vi "_caraya_updateVInames.vi"(8 "error in (no error)":errorcluster, 10 "Application":refnum<vi>, 11 "Class Path":path=path "C:/Projects/JKI/Caraya/src/tests/test-all-asserts/Test Runner.AllAsserts.lvclass") -> (0 "error out":errorcluster)   [LabVIEW 2013]
uses:
  <vilib>/regexp/Match Regular Expression.xnode
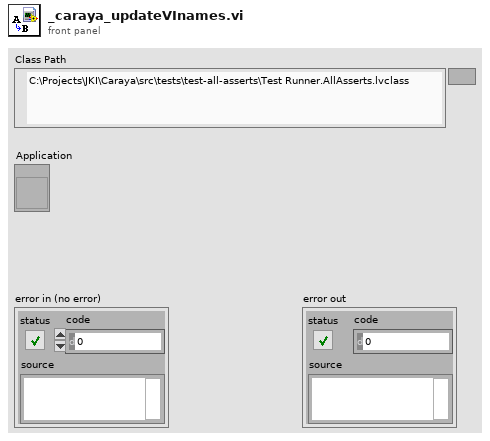
[diagram p1: front panel]
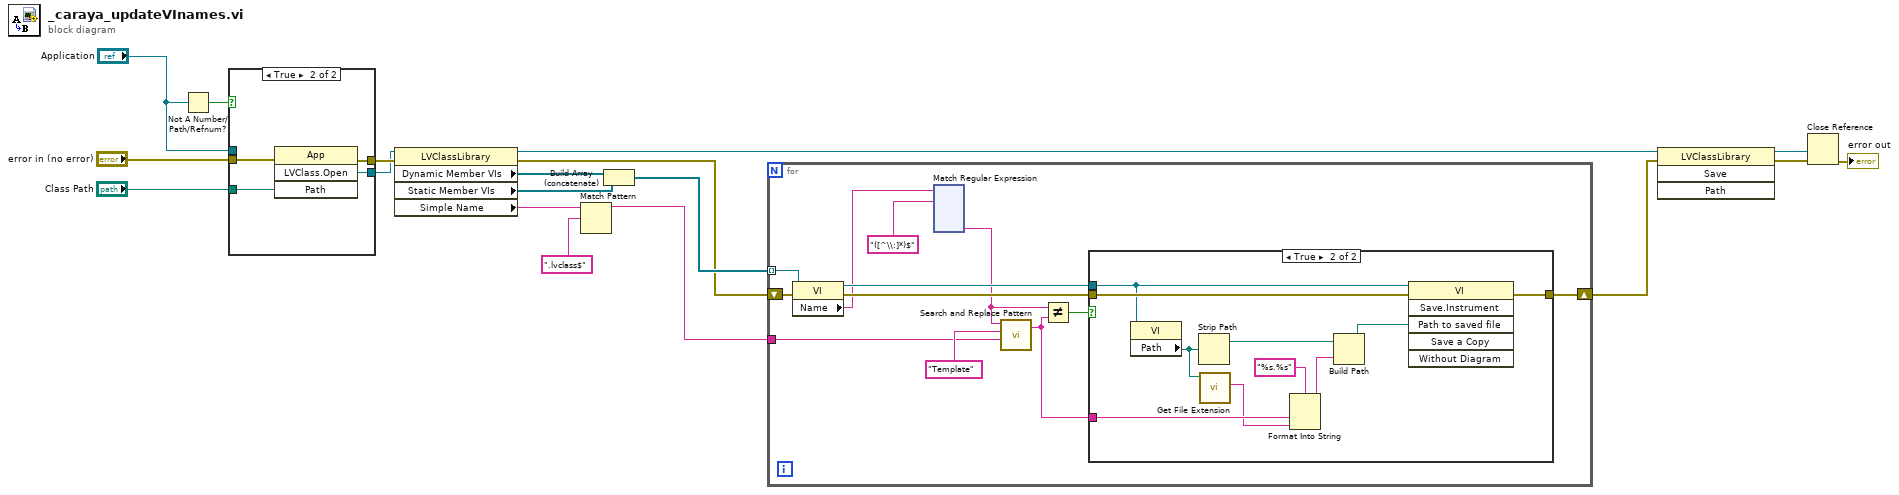
[diagram p0: block diagram]
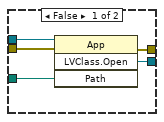
[diagram p2: hidden frame]
diagram:
  n1 = Not A Number/Path/Refnum?(number/path/refnum="Application") -> (NaN/Path/Refnum?=w4:bool)
  n2 = case shown="True" w4 {
    tunnel: [w23 w27] -> w13
    tunnel: [w22 w26] -> w11
    tunnel: "Class Path" -> [w21 w25]
    tunnel: "error in (no error)" -> [w20 w24]
    tunnel: "Application" -> [w19 _]
    frame False {
      n3 = invoke class="App" method="LVClass.Open"(reference=w19, error in=w20, "Path"=w21) -> (error out=w23:errorcluster, "LVClass.Open"=w22:refnum<vi>)  [unwired: 1 in, 2 out]
    }
    frame True {
      n4 = invoke class="App" method="LVClass.Open"(error in=w24, "Path"=w25) -> (error out=w27:errorcluster, "LVClass.Open"=w26:refnum<vi>)  [unwired: 2 in, 2 out]
    }
  }
  n5 = property class="LVClassLibrary"(reference=w11, error in=w13) -> (reference out=w12:refnum<vi>, error out=w9:errorcluster, "Dynamic Member VIs"=w18:refnum<vi>[], "Static Member VIs"=w17:refnum<vi>[], "Simple Name"=w2:string)
  n6 = Match Pattern(string=w2, regular expression=".lvclass$") -> (before substring=w1:string)  [unwired: 1 in, 3 out]
  n7 = Build Array (concatenate)(w18, w17) -> (w16:refnum<vi>[])
  n8 = for {
    tunnel: w16 -> [w32] mode=indexing
    shift-right: [w35] -> w8
    shift-left: w9 -> [w33]
    tunnel: w1 -> [w38]
    n9 = property class="VI"(reference=w32, error in=w33) -> (reference out=w36:refnum<vi>, error out=w34:errorcluster, "Name"=w30:string)
    n10 = xnode "Match Regular Expression"("input string"=w30, "regular expression"="([^\\:]*)$") -> ("submatch 1"=w29:string)  [unwired: 4 in, 5 out]
    n11 = call <vilib>:"Search and Replace Pattern.vi"("string"=w29, "regular expression (\"\")"="Template" ("regular expression"), "replace string (\"\")"=w38) -> ("result string"=w37:string)  [unwired: 2 in, 1 out]
    n12 = Not Equal?(x=w29, y=w37) -> (x != y?=w28:bool)
    n13 = case shown="True" w28 {
      tunnel: w36 -> [_ w164]
      tunnel: w37 -> [_ w161]
      tunnel: w34 -> [w156 w166]
      tunnel: [w156 w165] -> w35
      frame False {
      }
      frame True {
        n14 = property class="VI"(reference=w164) -> ("Path"=w162:path)  [unwired: 1 in, 2 out]
        n15 = Strip Path(path=w162) -> (stripped path=w163:path)  [unwired: 1 out]
        n16 = call <vilib>:"Get File Extension.vi"("file"=w162) -> ("lowercase file extension"=w160:string)  [unwired: 7 in, 3 out]
        n17 = Format Into String(format string="%s.%s", w161, w160) -> (resulting string=w158:string)  [unwired: 2 in, 1 out]
        n18 = Build Path(base path=w163, name or relative path=w158) -> (appended path=w157:path)
        n19 = invoke class="VI" method="Save.Instrument"(reference=w164, error in=w166, "Path to saved file"=w157) -> (error out=w165:errorcluster)  [unwired: 3 in, 5 out]
      }
    }
  }
  n20 = invoke class="LVClassLibrary" method="Save"(reference=w12, error in=w8) -> (reference out=w14:refnum<vi>, error out=w15:errorcluster)  [unwired: 2 in, 2 out]
  n21 = Close Reference(reference=w14, error in (no error)=w15) -> (error out=→"error out":errorcluster)
